vi "Translation_UnaryMinus.vi"(11 "In Translation":T1) -> (3 "Out Translation":T1)   [LabVIEW 2019, in "Trajectory_Library.lvlib"]
doc: "Returns the inverse of the current translation. This is equivalent to rotating by 180 degrees, flipping the point over both axes, or simply negating both components of the translation.\n \nParameters:\n - In Translation - This translation data structure\n\nResult:\n - Out Translation - The inverse of the current translation."
uses:
  Trajectory_Library.lvlib
  TRANSLATION2D.ctl
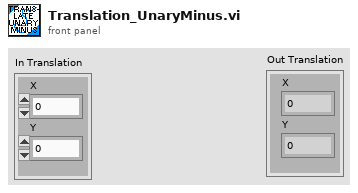
[diagram p1: front panel]
types:
  T1 = typedef "Trajectory_Library.lvlib/TRANSLATION2D.ctl" = cluster{"X":dbl, "Y":dbl}
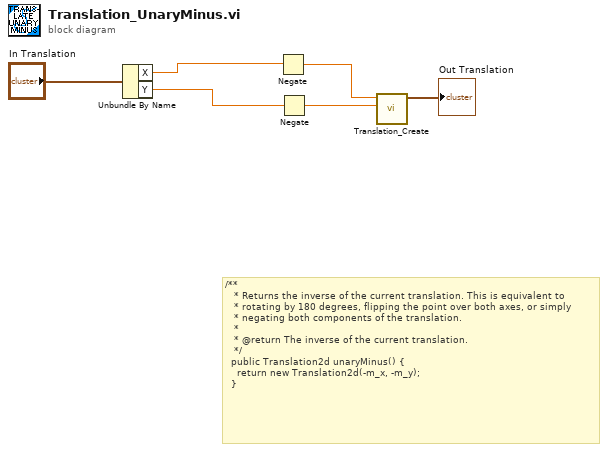
[diagram p0: block diagram]
diagram:
  # "/**\n   * Returns the inverse of the current translation. This is equivalent to\n   * rotating by 180 degrees, flipping the point over both axes, or simply\n   * negating both components of the translation.\n   *\n   * @return The inverse of the current translation.\n   */\n  public Translation2d unaryMinus() {\n    return new Translation2d(-m_x, -m_y);\n  }"
  n1 = Unbundle By Name("In Translation") -> ("X"=w4:dbl, "Y"=w2:dbl)
  n2 = Negate(x=w4) -> (-x=w3:dbl)
  n3 = Negate(x=w2) -> (-x=w1:dbl)
  n4 = call "Translation_Create.vi"("Y"=w1, "X"=w3) -> ("TRANSLATION"=→"Out Translation":T1)  [unwired: 9 in]
